vi "ImplementInterface.vi"(6 "InterfaceMethodsToCreate":string[](array[string])=["Add.Vi", "Execute.vi"], 7 "ClassWriter.lvclass":refnum<class "ClassWriter.lvclass">, 8 "error in":errorcluster, 9 "CreateMethods":bool=TRUE, 10 "Interface Path":path=path "C:/Projects/Interface/Sub_Interface1/Sub_Interface1.lvclass", 11 "LvClassPath/LvClassProjectItem":variant) -> (0 "error out":errorcluster={"status"=TRUE, "code"=7, "source"="Invoke Node in InterfaceLibrary.lvlib:ImplementInterface.vi\n<APPEND>\nMethod Name: <b>LabVIEW Class:Open</b>"})   [LabVIEW 2020, in "InterfaceLibrary.lvlib"]
uses:
  <resource>/Framework/Providers/Open_GDS/ClassProviders/Common/InterfaceLibrary/InterfaceLibrary.lvlib
  <resource>/Framework/Providers/Open_GDS/ClassProviders/Provider_BaseClassInterface/ClassWriter_class/ClassWriter.lvclass
  <resource>/Framework/Providers/Open_GDS/ClassProviders/Provider_LvNativeClass/ClassWriterNative_class/ClassWriterNative.lvclass
  <resource>/Framework/Providers/Open_GDS/API/GDSAPI_SubVIs/GDSAPI_MethodType.ctl
  <resource>/Framework/Providers/Open_GDS/ClassProviders/Provider_BaseClassInterface/CreateMethodData.ctl
  <resource>/Framework/Providers/Open_GDS/ClassProviders/Provider_EndevoGOOP300/GOOP300_SubVIs/GOOP300_MethodScopeType.ctl
  <resource>/Framework/Providers/Open_GDS/ClassProviders/Provider_LvNativeClass/ClassWriterNative_class/IconDetails.ctl
  <resource>/Framework/Providers/Open_GDS/ClassProviders/Provider_LvNativeClass/ClassWriterNative_class/IconSize.ctl
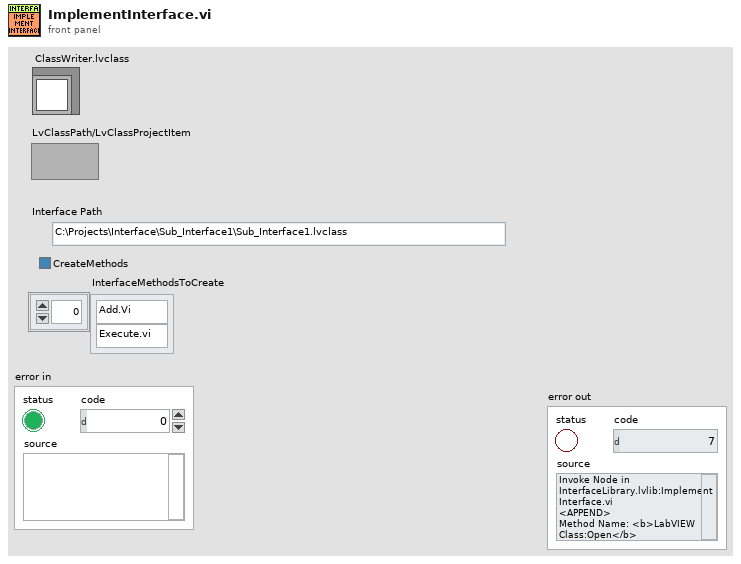
[diagram p1: front panel]
types:
  T1 = cluster{"ClassRef":refnum<vi>, "ClassRefCreated":bool, "Application":refnum<vi>, "InterfaceRef":refnum<vi>, "MethodsToImplement":path[], "MethodsDescription":string[], "MethodsScope":enum32{"invalid scope", "public", "private", "protected", "community"}[]}
  T2 = enum32{"invalid scope", "public", "private", "protected", "community"}
  T3 = typedef "GDSAPI_MethodType.ctl" = enum16{"Read Attribute", "Write Attribute", "Read & Write Attribute", "None Modifying Method", "Get Property", "Set Property", "Read Property", "Write Property", "Static Method", "Interface Method"}
  T4 = typedef "ClassWriter.lvclass/CreateMethodData.ctl" = cluster{"MethodName":string, "RelativeMethodPath":path, "MethodDescription":string, "Scope/Visibility":T5, "MethodTemplateName":string, "IconOut":u8[][], "RelativeProjectClassPath":string, "OpenViAfterCreation":bool, "DynamicDispatchVi":bool, "ExtraCreateParameters":variant, "MustOverride":bool, "MustCallParent":bool, "IconDetails":T6, "AF-Option":variant, "TemplatePath":path}
  T5 = typedef "GOOP300_MethodScopeType.ctl" = enum16{"Use Parent Folder Scope", "Public", "Protected", "Private", "Community"}
  T6 = typedef "ClassWriterNative.lvclass/IconDetails.ctl" = cluster{"IconSize":T7, "ImageRows(32)":i32, "ConnectorPaneHeight":i32[]}
  T7 = typedef "ClassWriterNative.lvclass/IconSize.ctl" = enum16{"Full", "1 c-term high", "2 c-term high", "3 c-term high"}
  T8 = enum32{"invalid scope", "public", "private", "protected", "community"}[]
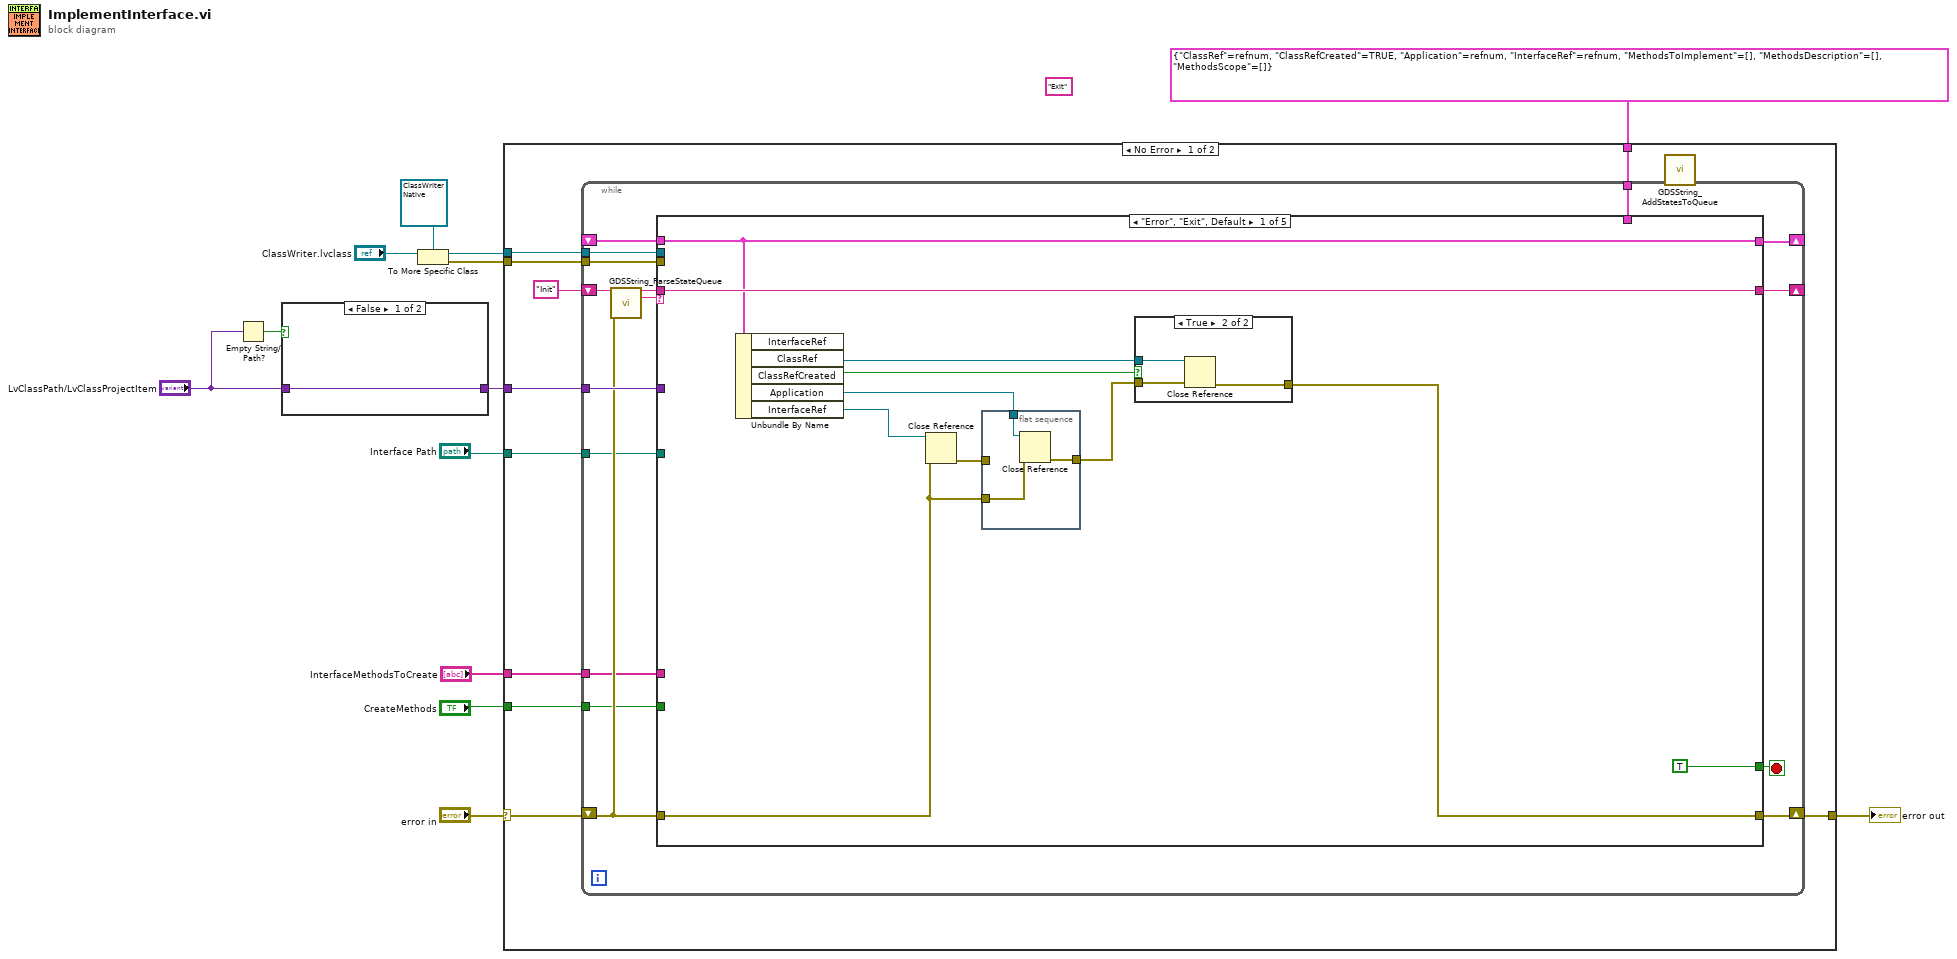
[diagram p0: block diagram]
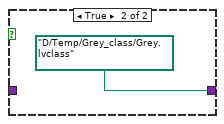
[diagram p2: hidden frame]
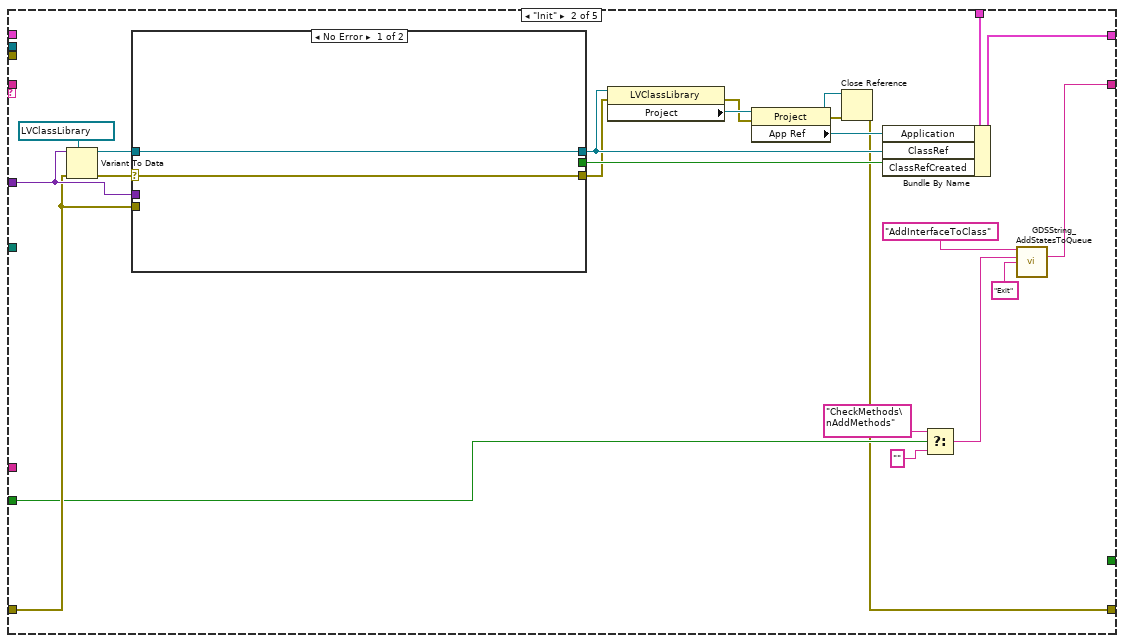
[diagram p4: hidden frame]
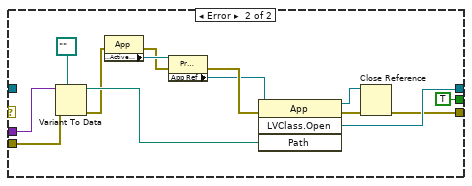
[diagram p5: hidden frame]
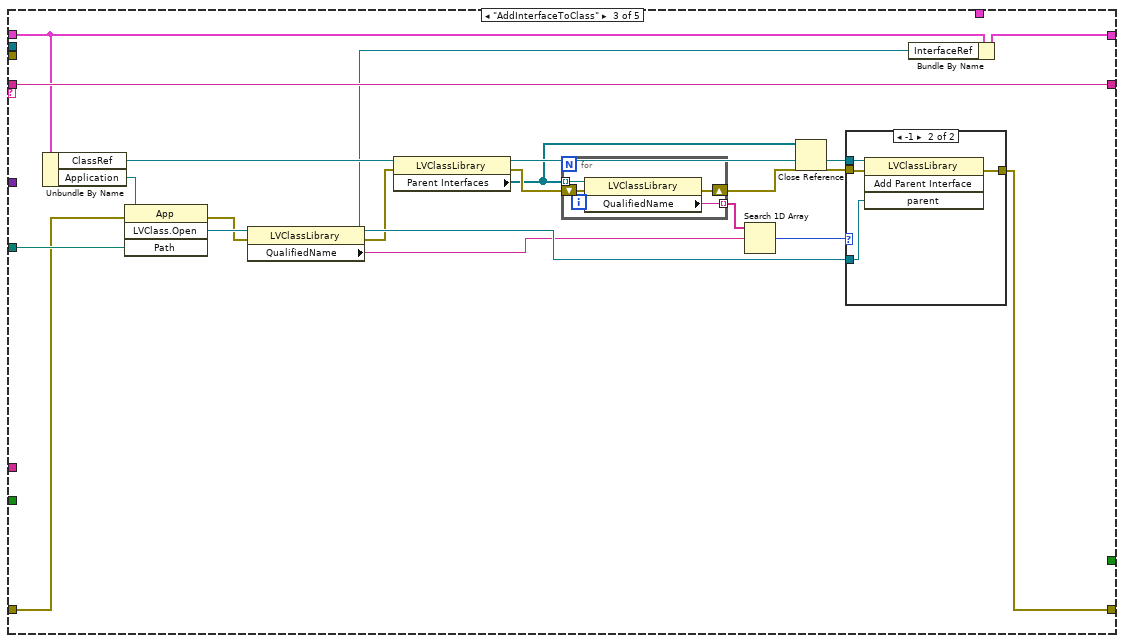
[diagram p6: hidden frame]
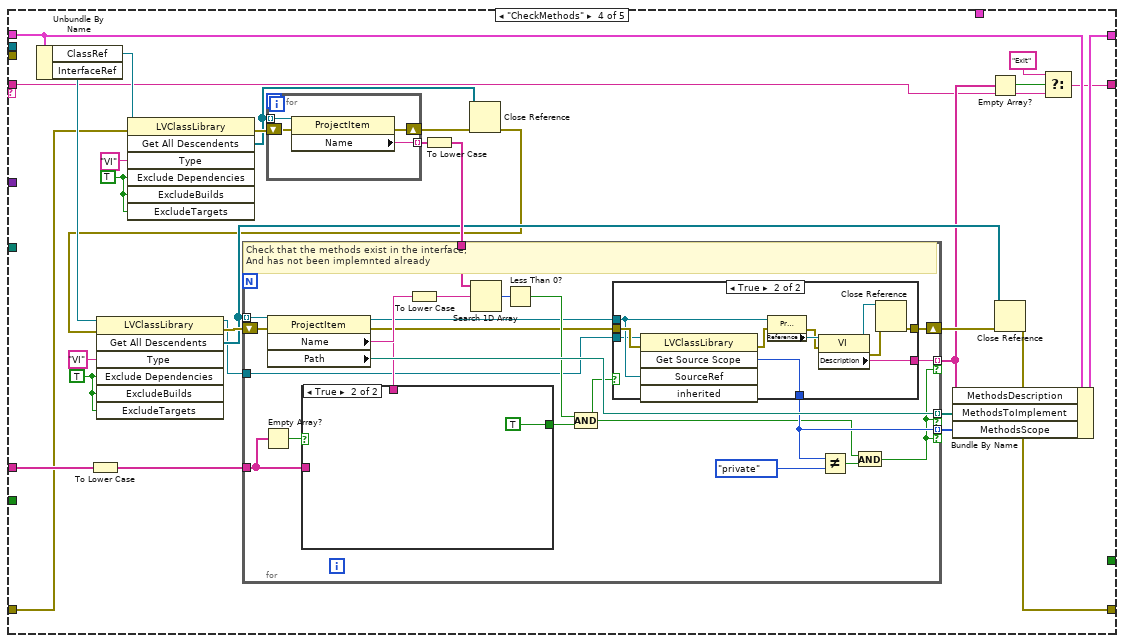
[diagram p8: hidden frame]
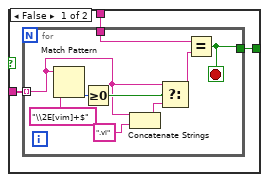
[diagram p10: hidden frame]
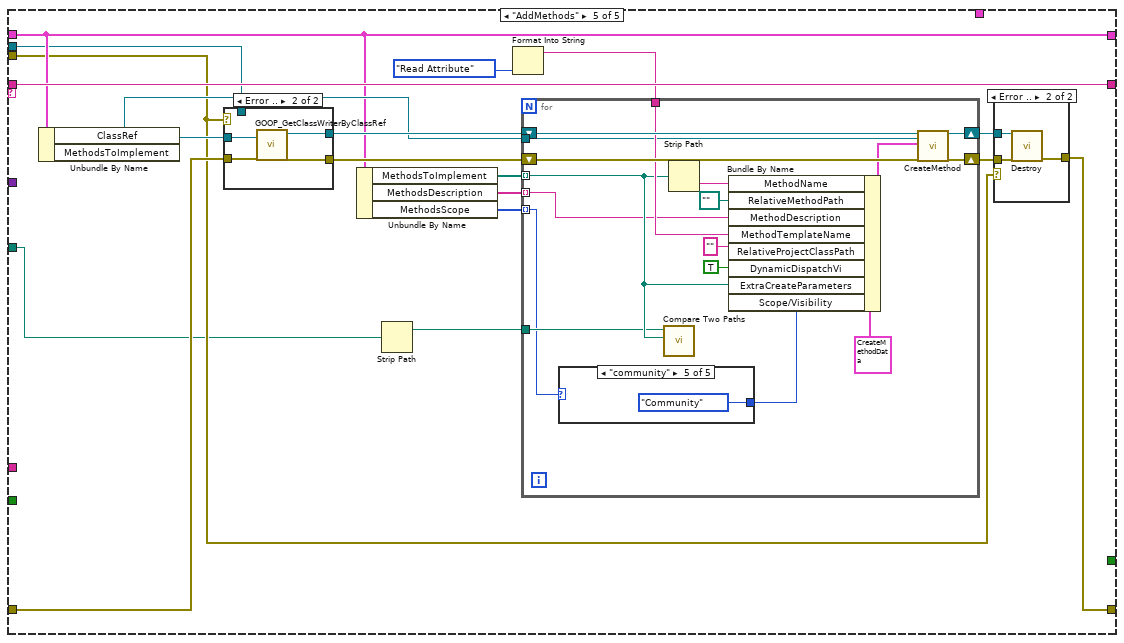
[diagram p11: hidden frame]
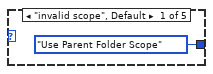
[diagram p14: hidden frame]
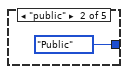
[diagram p15: hidden frame]
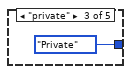
[diagram p16: hidden frame]
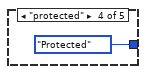
[diagram p17: hidden frame]
diagram:
  (unwired) "Exit" ("Remaining States")
  n1 = Empty String/Path?(string/path="LvClassPath/LvClassProjectItem") -> (empty?=w9:bool)
  n2 = case shown="False" w9 {
    tunnel: "LvClassPath/LvClassProjectItem" -> [w14 _]
    tunnel: [w14 path "D:/Temp/Grey_class/Grey.lvclass" ("Path")] -> w7
    frame False {
    }
    frame True {
    }
  }
  n3 = To More Specific Class(target class=refnum<class "ClassWriterNative.lvclass"> refnum ("ClassWriterNative"), reference="ClassWriter.lvclass") -> (specific class reference=w3:refnum<class "ClassWriterNative.lvclass">, error out=w1:errorcluster)  [unwired: 1 in]
  n4 = case shown="No Error" "error in" {
    selector: "error in" -> [w24 w257]
    tunnel: w7 -> [w25 _]
    tunnel: [w23 w257] -> w12
    tunnel: T1 {"ClassRef"=refnum, "ClassRefCreated"=TRUE, "Application"=refnum, "InterfaceRef"=refnum, "MethodsToImplement"=[], "MethodsDescription"=[], "MethodsScope"=[]} -> [w21 _]
    tunnel: "CreateMethods" -> [w20 _]
    tunnel: "Interface Path" -> [w19 _]
    tunnel: "InterfaceMethodsToCreate" -> [w18 _]
    tunnel: w3 -> [w17 _]
    tunnel: w1 -> [w16 _]
    frame No Error {
      n5 = while {
        tunnel: w25 -> [w41]
        shift-right: [w40] -> w23
        shift-left: w24 -> [w38]
        shift-right: [w32] -> _
        shift-left: "Init" -> [w39]
        tunnel: w21 -> [w36]
        shift-right: [w35] -> _
        shift-left: _ -> [w34]
        tunnel: w20 -> [w30]
        tunnel: w19 -> [w29]
        tunnel: w18 -> [w28]
        tunnel: w17 -> [w27]
        tunnel: w16 -> [w26]
        stop <- w31 stop-if-true
        n6 = call <resource>:"GDSString_ParseStateQueue.vi"("State Queue"=w39, "Error In (no error)"=w38) -> ("Remaining States"=w33:string, "Current State"=w37:string)  [unwired: 9 in, 3 out]
        n7 = case shown="\"Error\", \"Exit\", Default" w37 {
          tunnel: w41 -> [_ w79 _ _ _]
          tunnel: w38 -> [w42 w78 w110 w135 w215]
          tunnel: [w45 w62 w111 w136 w219] -> w40
          tunnel: [w50 w76 w109 w145 w213] -> w35
          tunnel: w36 -> [_ w77 _ _ _]
          tunnel: w34 -> [w50 _ w117 w154 w213]
          tunnel: [w52 w74 w118 w143 w224] -> w32
          tunnel: w33 -> [w52 _ w118 w132 w224]
          tunnel: [TRUE _ _ _ _] -> w31
          tunnel: w30 -> [_ w73 _ _ _]
          tunnel: w29 -> [_ _ w114 _ w207]
          tunnel: w28 -> [_ _ _ w149 _]
          tunnel: w27 -> [_ _ _ _ w209]
          tunnel: w26 -> [_ _ _ _ w210]
          frame "Error", "Exit", Default {
            n8 = Unbundle By Name(w50) -> ("ClassRef"=w48:refnum<vi>, "ClassRefCreated"=w49:bool, "Application"=w47:refnum<vi>, "InterfaceRef"=w44:refnum<vi>)  [unwired: 1 out]
            n9 = Close Reference(reference=w44, error in (no error)=w42) -> (error out=w43:errorcluster)
            n10 = flat-sequence {
              tunnel: w47 -> [w55]
              tunnel: [w54] -> w46
              tunnel: w43 -> [_]
              tunnel: w42 -> [w53]
              frame #0 {
                n11 = Close Reference(reference=w55, error in (no error)=w53) -> (error out=w54:errorcluster)
              }
            }
            n12 = case shown="True" w49 {
              tunnel: w48 -> [_ w59]
              tunnel: w46 -> [w56 w58]
              tunnel: [w56 w57] -> w45
              frame False {
              }
              frame True {
                n13 = Close Reference(reference=w59, error in (no error)=w58) -> (error out=w57:errorcluster)
              }
            }
          }
          frame "Init" {
            n14 = Variant To Data(error in=w78, type=refnum<vi> refnum ("ProjectItem"), Variant=w79) -> (data=w81:refnum<vi>, error out=w80:errorcluster)
            n15 = case shown="No Error" w80 {
              selector: w80 -> [w83 _]
              tunnel: w81 -> [w84 _]
              tunnel: [w83 w90] -> w63
              tunnel: w79 -> [_ w97]
              tunnel: w78 -> [_ w94]
              tunnel: [w84 w93] -> w67
              tunnel: [_ TRUE] -> w75
              frame No Error {
              }
              frame Error {
                n16 = Variant To Data(error in=w94, type=path "" ("Path"), Variant=w97) -> (data=w96:path, error out=w95:errorcluster)
                n17 = property class="App"(error in=w95) -> (error out=w87:errorcluster, "Project.ActiveProject"=w88:refnum<vi>)  [unwired: 1 in, 1 out]
                n18 = property class="Project"(reference=w88, error in=w87) -> (error out=w86:errorcluster, "App Ref"=w85:refnum<vi>)  [unwired: 1 out]
                n19 = invoke class="App" method="LVClass.Open"(reference=w85, error in=w86, "Path"=w96) -> (reference out=w91:refnum<vi>, error out=w92:errorcluster, "LVClass.Open"=w93:refnum<vi>)  [unwired: 1 in, 1 out]
                n20 = Close Reference(reference=w91, error in (no error)=w92) -> (error out=w90:errorcluster)
              }
            }
            n21 = property class="LVClassLibrary"(reference=w67, error in=w63) -> (error out=w60:errorcluster, "Project"=w61:refnum<vi>)  [unwired: 1 out]
            n22 = property class="Project"(reference=w61, error in=w60) -> (reference out=w65:refnum<vi>, error out=w64:errorcluster, "App Ref"=w66:refnum<vi>)
            n23 = Close Reference(reference=w65, error in (no error)=w64) -> (error out=w62:errorcluster)
            n24 = Bundle By Name(cluster=w77, "Application"=w66, "ClassRef"=w67, "ClassRefCreated"=w75) -> (w76:T1)
            n25 = Select(t="CheckMethods\nAddMethods" ("Remaining States"), s=w73, f="") -> (s? t:f=w69:string)
            n26 = call <resource>:"GDSString_AddStatesToQueue.vi"("State(s) in Front (\"\")"="AddInterfaceToClass" ("Remaining States"), "State(s) in (\"\")"=w69, "State(s) at Back (\"\")"="Exit" ("Remaining States")) -> ("States Out"=w74:string)  [unwired: 12 in]
          }
          frame "AddInterfaceToClass" {
            n27 = Unbundle By Name(w117) -> ("ClassRef"=w116:refnum<vi>, "Application"=w115:refnum<vi>)
            n28 = invoke class="App" method="LVClass.Open"(reference=w115, error in=w110, "Path"=w114) -> (error out=w105:errorcluster, "LVClass.Open"=w108:refnum<vi>)  [unwired: 1 in, 2 out]
            n29 = property class="LVClassLibrary"(reference=w108, error in=w105) -> (reference out=w107:refnum<vi>, error out=w104:errorcluster, "QualifiedName"=w106:string)
            n30 = property class="LVClassLibrary"(reference=w116, error in=w104) -> (reference out=w112:refnum<vi>, error out=w103:errorcluster, "Parent Interfaces"=w99:refnum<vi>[])
            n31 = for {
              tunnel: w99 -> [w122] mode=indexing
              tunnel: [w121] -> w102 mode=indexing
              shift-right: [w120] -> w101
              shift-left: w103 -> [w119]
              n32 = property class="LVClassLibrary"(reference=w122, error in=w119) -> (error out=w120:errorcluster, "QualifiedName"=w121:string)  [unwired: 1 out]
            }
            n33 = Search 1D Array(1D array=w102, element=w106) -> (index of element=w113:i32)  [unwired: 1 in]
            n34 = Close Reference(reference=w99, error in (no error)=w101) -> (error out=w100:errorcluster)
            n35 = case shown="-1" w113 {
              tunnel: w112 -> [_ w127]
              tunnel: w100 -> [w123 w126]
              tunnel: w107 -> [_ w125]
              tunnel: [w123 w124] -> w111
              frame 0, Default {
              }
              frame -1 {
                n36 = invoke class="LVClassLibrary" method="Add Parent Interface"(reference=w127, error in=w126, "parent"=w125) -> (error out=w124:errorcluster)  [unwired: 1 in, 3 out]
              }
            }
            n37 = Bundle By Name(cluster=w117, "InterfaceRef"=w107) -> (w109:T1)
          }
          frame "CheckMethods" {
            w152 = TRUE ("ExcludeDependencies")
            w155 = TRUE ("ExcludeDependencies")
            n38 = Unbundle By Name(w154) -> ("ClassRef"=w153:refnum<vi>, "InterfaceRef"=w150:refnum<vi>)
            n39 = To Lower Case(string=w149) -> (all lower case string=w148:string[])
            n40 = invoke class="LVClassLibrary" method="Get All Descendents"(reference=w153, error in=w135, "Type"="VI", "Exclude Dependencies"=w155, "ExcludeBuilds"=w155, "ExcludeTargets"=w155) -> (error out=w156:errorcluster, "All Descendents"=w137:refnum<vi>[])  [unwired: 1 in, 5 out]
            n41 = for {
              tunnel: w137 -> [w206] mode=indexing
              tunnel: [w205] -> w147 mode=indexing
              shift-right: [w203] -> w139
              shift-left: w156 -> [w204]
              n42 = property class="ProjectItem"(reference=w206, error in=w204) -> (error out=w203:errorcluster, "Name"=w205:string)  [unwired: 1 out]
            }
            n43 = To Lower Case(string=w147) -> (all lower case string=w146:string[])
            n44 = Close Reference(reference=w137, error in (no error)=w139) -> (error out=w138:errorcluster)
            n45 = invoke class="LVClassLibrary" method="Get All Descendents"(reference=w150, error in=w138, "Type"="VI", "Exclude Dependencies"=w152, "ExcludeBuilds"=w152, "ExcludeTargets"=w152) -> (reference out=w130:refnum<vi>, error out=w151:errorcluster, "All Descendents"=w140:refnum<vi>[])  [unwired: 1 in, 4 out]
            n46 = for {
              tunnel: w140 -> [w177] mode=indexing
              shift-right: [w164] -> w141
              shift-left: w151 -> [w176]
              tunnel: [w175] -> w134 mode=indexing if=w157
              tunnel: w148 -> [w173]
              tunnel: w146 -> [w169]
              tunnel: [w163] -> w133 mode=indexing if=w157
              tunnel: [w161] -> w131 mode=indexing if=w157
              tunnel: w130 -> [w162]
              # "Check that the methods exist in the interface,\nAnd has not been implemnted already"
              n47 = Empty Array?(array=w173) -> (empty?=w171:bool)
              n48 = property class="ProjectItem"(reference=w177, error in=w176) -> (reference out=w165:refnum<vi>, error out=w166:errorcluster, "Name"=w174:string, "Path"=w175:path)
              n49 = To Lower Case(string=w174) -> (all lower case string=w170:string)
              n50 = case shown="True" w171 {
                tunnel: w170 -> [w192 _]
                tunnel: w173 -> [w191 _]
                tunnel: [w190 TRUE] -> w172
                frame False {
                  n51 = for {
                    tunnel: [w193] -> w190
                    tunnel: w192 -> [w196]
                    tunnel: w191 -> [w195] mode=indexing
                    stop <- w193 stop-if-true
                    n52 = Match Pattern(string=w195, regular expression="\\2E[vim]+$") -> (offset past match=w200:i32)  [unwired: 1 in, 3 out]
                    n53 = Greater Or Equal To 0?(x=w200) -> (x >= 0?=w199:bool)
                    n54 = Concatenate Strings(w195, ".vi" ("string")) -> (w198:string)
                    n55 = Select(t=w195, s=w199, f=w198) -> (s? t:f=w194:string)
                    n56 = Equal?(x=w196, y=w194) -> (x = y?=w193:bool)
                  }
                }
                frame True {
                }
              }
              n57 = Search 1D Array(1D array=w169, element=w170) -> (index of element=w168:i32)  [unwired: 1 in]
              n58 = Less Than 0?(x=w168) -> (x < 0?=w167:bool)
              n59 = Compound Arithmetic op=AND(w167, w172) -> (w158:bool)
              n60 = case shown="True" w158 {
                tunnel: w166 -> [w178 w182]
                tunnel: w165 -> [_ w181]
                tunnel: [w178 w184] -> w164
                tunnel: [_ w187] -> w163
                tunnel: [_ w180] -> w161
                tunnel: w162 -> [_ w179]
                frame False {
                }
                frame True {
                  n61 = invoke class="LVClassLibrary" method="Get Source Scope"(reference=w179, error in=w182, "SourceRef"=w181) -> (error out=w183:errorcluster, "GetSourceScope"=w180:T2)  [unwired: 2 in, 3 out]
                  n62 = property class="ProjectItem"(reference=w181, error in=w183) -> (error out=w188:errorcluster, "Reference"=w189:refnum<vi>)  [unwired: 1 out]
                  n63 = property class="VI"(reference=w189, error in=w188) -> (reference out=w186:refnum<vi>, error out=w185:errorcluster, "Description"=w187:string)
                  n64 = Close Reference(reference=w186, error in (no error)=w185) -> (error out=w184:errorcluster)
                }
              }
              n65 = Not Equal?(x=w161, y=T2."private") -> (x != y?=w159:bool)
              n66 = And(x=w158, y=w159) -> (x .and. y?=w157:bool)
            }
            n67 = Bundle By Name(cluster=w154, "MethodsDescription"=w133, "MethodsToImplement"=w134, "MethodsScope"=w131) -> (w145:T1)
            n68 = Empty Array?(array=w133) -> (empty?=w144:bool)
            n69 = Close Reference(reference=w140, error in (no error)=w141) -> (error out=w136:errorcluster)
            n70 = Select(t="Exit" ("Remaining States"), s=w144, f=w132) -> (s? t:f=w143:string)
          }
          frame "AddMethods" {
            n71 = Unbundle By Name(w213) -> ("ClassRef"=w216:refnum<vi>)  [unwired: 1 out]
            n72 = case shown="Error .." w210 {
              tunnel: w216 -> [_ w234]
              tunnel: [w230 w233] -> w223
              tunnel: [w229 w232] -> w222
              tunnel: w209 -> [w230 _]
              tunnel: w215 -> [w229 w231]
              frame No Error {
              }
              frame Error {
                n73 = call <resource>:"GOOP_GetClassWriterByClassRef.vi"("LVClassLibrary Refnum"=w234, "error in (no error)"=w231) -> ("ClassWriterNative.lvclass"=w233:refnum<class "ClassWriterNative.lvclass">, "error out"=w232:errorcluster)  [unwired: 16 in]
              }
            }
            n74 = Unbundle By Name(w213) -> ("MethodsToImplement"=w214:path[], "MethodsDescription"=w212:string[], "MethodsScope"=w211:T8)
            n75 = Strip Path(path=w207) -> (stripped path=w208:path)  [unwired: 1 out]
            n76 = Format Into String(GDSAPI_MethodType."Read Attribute" ("MethodType")) -> (resulting string=w217:string)  [unwired: 3 in, 1 out]
            n77 = for {
              shift-right: [w249] -> w221
              shift-left: w223 -> [w251]
              shift-right: [w248] -> w220
              shift-left: w222 -> [w250]
              tunnel: w217 -> [w247]
              tunnel: w214 -> [w246] mode=indexing
              tunnel: w208 -> [w245]
              tunnel: w216 -> [w244]
              tunnel: w212 -> [w238] mode=indexing
              tunnel: w211 -> [w237] mode=indexing
              n78 = case shown="\"community\"" w237 {
                tunnel: [GOOP300_MethodScopeType."Use Parent Folder Scope" ("Scope/Visibility") GOOP300_MethodScopeType."Public" ("Scope/Visibility") GOOP300_MethodScopeType."Private" ("Scope/Visibility") GOOP300_MethodScopeType."Protected" ("Scope/Visibility") GOOP300_MethodScopeType."Community" ("Scope/Visibility")] -> w236
                frame "invalid scope", Default {
                }
                frame "public" {
                }
                frame "private" {
                }
                frame "protected" {
                }
                frame "community" {
                }
              }
              n79 = call <vilib>:"Compare Two Paths.vi"("Path 2"=w246, "Path 1"=w245) -> ()  [unwired: 6 in, 4 out]
              n80 = Strip Path(path=w246) -> (name=w240:string)  [unwired: 1 out]
              n81 = Bundle By Name(cluster=T4 {"MethodName"="", "RelativeMethodPath"=path "", "MethodDescription"="", "Scope/Visibility"=enum."Use Parent Folder Scope", "MethodTemplateName"="", "IconOut"=[], "RelativeProjectClassPath"="", "OpenViAfterCreation"=FALSE, "DynamicDispatchVi"=FALSE, "ExtraCreateParameters"=variant, "MustOverride"=FALSE, "MustCallParent"=FALSE, "IconDetails"={"IconSize"=enum."Full", "ImageRows(32)"=0, "ConnectorPaneHeight"=[]}, "AF-Option"=variant, "TemplatePath"=path ""} ("CreateMethodData"), "MethodName"=w240, "RelativeMethodPath"=path "", "MethodDescription"=w238, "MethodTemplateName"=w247, "RelativeProjectClassPath"="", "DynamicDispatchVi"=TRUE, "ExtraCreateParameters"=w246, "Scope/Visibility"=w236) -> (w241:T4)
              n82 = call-dynamic "CreateMethod.vi"("ClassWriterNative.lvclass"=w251, "ClassItemRefIn"=w244, "CreateMethodData"=w241, "error in (no error)"=w250) -> ("ClassWriterNative.lvclass 2"=w249:refnum<class "ClassWriterNative.lvclass">, "error out"=w248:errorcluster)  [unwired: 12 in, 2 out]
            }
            n83 = case shown="Error .." w210 {
              tunnel: w221 -> [_ w228]
              tunnel: w220 -> [w225 w227]
              tunnel: [w225 w226] -> w219
              frame No Error {
              }
              frame Error {
                n84 = call-dynamic "Destroy.vi"("ClassWriterNative"=w228, "error in (no error)"=w227) -> ("error out"=w226:errorcluster)  [unwired: 17 in]
              }
            }
          }
        }
      }
      n85 = call <resource>:"GDSString_AddStatesToQueue.vi"() -> ()  [unwired: 15 in, 1 out]
    }
    frame Error {
    }
  }
  "error out" <- w12
